vi "Exp_CCD_GetExposureTime.vi"(8 "error in (no error)":errorcluster, 11 "LightField Automation in":refnum<class "LightField Automation.lvclass">) -> (0 "error out":errorcluster, 2 "Exposure Time (s)":dbl, 3 "LightField Automation out":refnum<class "LightField Automation.lvclass">)   [LabVIEW 2015, in "LightField Automation.lvclass"]
uses:
  LightField Automation.lvclass
  C:/Program Files/Princeton Instruments/LightField/PrincetonInstruments.LightFieldAddInSupportServices.dll
  Program Files/Princeton Instruments/LightField/PrincetonInstruments.LightFieldAddInSupportServices.dll
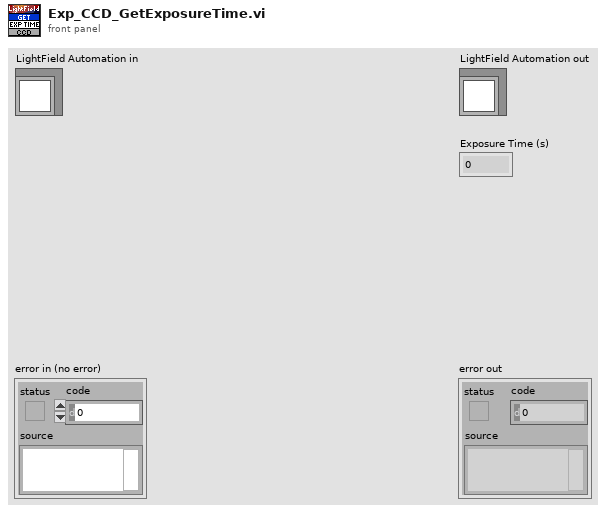
[diagram p1: front panel]
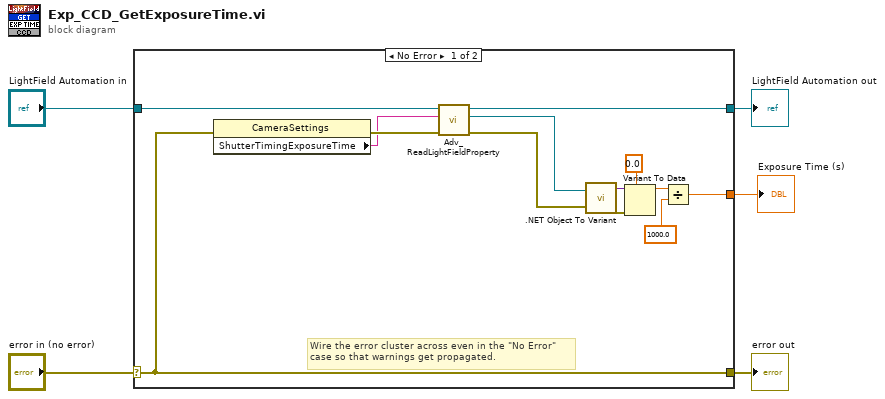
[diagram p0: block diagram]
diagram:
  n1 = case shown="No Error" "error in (no error)" {
    selector: "error in (no error)" -> [w13 w20]
    tunnel: [w13 w20] -> w4
    tunnel: [w10 w19] -> w2
    tunnel: "LightField Automation in" -> [w11 w19]
    tunnel: [w12 _] -> w1
    frame No Error {
      # "Wire the error cluster across even in the \"No Error\"\ncase so that warnings get propagated."
      n2 = property class="CameraSettings"(error in=w13) -> (error out=w9:errorcluster, "ShutterTimingExposureTime"=w8:string)  [unwired: 1 in, 1 out]
      n3 = call "Adv_ReadLightFieldProperty.vi"("error in (no error)"=w9, "setting"=w8, "LightField Automation in"=w11) -> ("error out"=w6:errorcluster, "value"=w7:refnum<k24>, "LightField Automation out"=w10:refnum<class "LightField Automation.lvclass">)  [unwired: 6 in]
      n4 = call <vilib>:".NET Object To Variant.vi"("error in (no error)"=w6, ".NET object"=w7) -> ("error out"=w16:errorcluster, "variant"=w14:variant)
      n5 = Variant To Data(error in=w16, type=0.0, Variant=w14) -> (data=w17:dbl)  [unwired: 1 out]
      n6 = Divide(x=w17, y=1000.0) -> (x/y=w12:dbl)
    }
    frame Error {
    }
  }
  "error out" <- w4
  "LightField Automation out" <- w2
  "Exposure Time (s)" <- w1
